vi "Pump Status.vi"(8 "error in (no error)":errorcluster, 11 "State in":T1={"State"=enum."Idle", "Start Time"=timestamp(0 s since 1904-01-01), "Configuration"={"Cycle Period"=0.0, "Ismatech"={"VISA resource name"="", "Simulated?"=FALSE, "Pump Number"=1.0, "Reverse?"=FALSE}, "Masterflex"={"VISA resource name"="", "Simulated?"=FALSE, "Pump Number"=1.0, "Reverse?"=FALSE}, "Mettler"={"VISA resource name"="", "Simulated?"=FALSE}, "Bronkhorst M13 Flow Meter"={"VISA resource name"="", "Simulated?"=FALSE, "Smoothing Steps"=1}, "PID 2 Parameters"={"Input Device"=enum."Bronkhorst M13", "Output Device"=enum."Ismatec ISM 831C", "Setpoint"=0.0, "PID gains"={"proportional gain (Kc)"=1.0, "integral time (Ti, min)"=0.01, "derivative time (Td, min)"=0.0}}, "Manual Entry"=0.0, "Auto?"=TRUE, "PID range"={"PID High"=100.0, "PID Low"=0.0, "High Warning"=100.0}, "Tacmina Settings"={"Analog DAQ Task"="", "Digital DAQ Task"=""}, "KNF SIMDOS Settings"={"VISA resource name"="", "Simulated?"=TRUE}, "ASIA Pump C"={"ASIA Pump #"=0, "channel"=0, "Simulated"=FALSE}, "VICI Settings"={"VISA resource name"="", "Pump ID"="", "Pump Head Vol"=0.0, "Reverse?"=FALSE, "Simulated?"=FALSE}, "FLOM Settings"={"VISA resource name"="", "Simulated?"=TRUE, "Pump Number"=0.0}, "SSI PR/LD Settings"={"VISA resource name"="", "Simulated?"=FALSE}, "Masterflex 75211 Settings"={"Analog DAQ Task"="", "Digital DAQ Task"=""}, "SSI P40 Settings"={"VISA resource name"="", "Simulated?"=TRUE}, "Ismatech 3 Channel Settings"={"VISA resource name"="", "Pump Number"=1, "Channel Number"=0, "Simulated?"=TRUE, "Reverse?"=FALSE}, "Bronkhorst M14 Settings"={"VISA resource name"="", "Simulated?"=FALSE, "Smoothing Steps"=1}, "Reset Totalizer"=FALSE, "Input Num Alarm Settings"=[], "Control Type"=enum."g/min", "Front End Display Options"={"Temperature"=TRUE, "Scale Grams"=FALSE, "Density"=TRUE, "Flow (g/min)"=FALSE, "Flow (ml/min)"=TRUE, "PSIG"=TRUE, "Total Grams"=TRUE, "Updated"=TRUE}}, "Current Time"=timestamp(0 s since 1904-01-01), "PID 1 Parameters"={"Setpoint"=0.0, "PID gains"={"proportional gain (Kc)"=1.0, "integral time (Ti, min)"=0.01, "derivative time (Td, min)"=0.0}}, "First Iteration"=FALSE, "Data"={"Flowmeter (g/min)"=0.0, "Flowmeter (ml/min)"=0.0, "Density"=0.0, "FL Temp"=0.0, "Scale Output (g)"=0.0, "Scale Rate of Change (g/min)"=0.0, "PID 1 Output"=0.0, "PID 2 Process Variable"=0.0, "PID 2 output"=0.0, "Pump Flow"=0.0, "Pump Pressure"=0.0, "Totalized Value"=0.0}, "Process Name"="", "Pump On?"=enum."Off", "Input Error"=FALSE, "Output Error"=FALSE, "Log Started"=FALSE, "PID Overshoot"=FALSE, "Current Setpoint"=0.0} {"PID 1 Parameters"."PID gains"."derivative time (Td, min)" format="%.3f"; "PID 1 Parameters"."PID gains"."integral time (Ti, min)" format="%.3f"; "PID 1 Parameters"."PID gains"."proportional gain (Kc)" format="%.3f"; "Configuration"."Bronkhorst M14 Settings"."Smoothing Steps" min=1 step=1; "Configuration"."Ismatech 3 Channel Settings"."Channel Number" min=0 max=3; "Configuration"."Ismatech 3 Channel Settings"."Pump Number" min=1; "Configuration"."PID range"."PID Low" min=0.0 max=100.0 format="%.2f"; "Configuration"."PID range"."PID High" format="%.2f"; "Configuration"."PID 2 Parameters"."PID gains"."derivative time (Td, min)" format="%.3f"; "Configuration"."PID 2 Parameters"."PID gains"."integral time (Ti, min)" format="%.3f"; "Configuration"."PID 2 Parameters"."PID gains"."proportional gain (Kc)" format="%.3f"; "Configuration"."Bronkhorst M13 Flow Meter"."Smoothing Steps" min=1 step=1; "Configuration"."ASIA Pump C"."channel" min=0 max=1 step=1; "Configuration"."Ismatech"."Pump Number" min=1.0 max=20.0 step=1.0; "Configuration"."Masterflex"."Pump Number" min=1.0 max=20.0 step=1.0}) -> (0 "error out":errorcluster, 3 "State out":T1={"State"=enum."Idle", "Start Time"=timestamp(0 s since 1904-01-01), "Configuration"={"Cycle Period"=0.0, "Ismatech"={"VISA resource name"="", "Simulated?"=FALSE, "Pump Number"=1.0, "Reverse?"=FALSE}, "Masterflex"={"VISA resource name"="", "Simulated?"=FALSE, "Pump Number"=1.0, "Reverse?"=FALSE}, "Mettler"={"VISA resource name"="", "Simulated?"=FALSE}, "Bronkhorst M13 Flow Meter"={"VISA resource name"="", "Simulated?"=FALSE, "Smoothing Steps"=1}, "PID 2 Parameters"={"Input Device"=enum."Bronkhorst M13", "Output Device"=enum."Ismatec ISM 831C", "Setpoint"=0.0, "PID gains"={"proportional gain (Kc)"=1.0, "integral time (Ti, min)"=0.01, "derivative time (Td, min)"=0.0}}, "Manual Entry"=0.0, "Auto?"=TRUE, "PID range"={"PID High"=100.0, "PID Low"=0.0, "High Warning"=100.0}, "Tacmina Settings"={"Analog DAQ Task"="", "Digital DAQ Task"=""}, "KNF SIMDOS Settings"={"VISA resource name"="", "Simulated?"=TRUE}, "ASIA Pump C"={"ASIA Pump #"=0, "channel"=0, "Simulated"=FALSE}, "VICI Settings"={"VISA resource name"="", "Pump ID"="", "Pump Head Vol"=0.0, "Reverse?"=FALSE, "Simulated?"=FALSE}, "FLOM Settings"={"VISA resource name"="", "Simulated?"=TRUE, "Pump Number"=0.0}, "SSI PR/LD Settings"={"VISA resource name"="", "Simulated?"=FALSE}, "Masterflex 75211 Settings"={"Analog DAQ Task"="", "Digital DAQ Task"=""}, "SSI P40 Settings"={"VISA resource name"="", "Simulated?"=TRUE}, "Ismatech 3 Channel Settings"={"VISA resource name"="", "Pump Number"=1, "Channel Number"=0, "Simulated?"=TRUE, "Reverse?"=FALSE}, "Bronkhorst M14 Settings"={"VISA resource name"="", "Simulated?"=FALSE, "Smoothing Steps"=1}, "Reset Totalizer"=FALSE, "Input Num Alarm Settings"=[], "Control Type"=enum."g/min", "Front End Display Options"={"Temperature"=TRUE, "Scale Grams"=FALSE, "Density"=TRUE, "Flow (g/min)"=FALSE, "Flow (ml/min)"=TRUE, "PSIG"=TRUE, "Total Grams"=TRUE, "Updated"=TRUE}}, "Current Time"=timestamp(0 s since 1904-01-01), "PID 1 Parameters"={"Setpoint"=0.0, "PID gains"={"proportional gain (Kc)"=1.0, "integral time (Ti, min)"=0.01, "derivative time (Td, min)"=0.0}}, "First Iteration"=FALSE, "Data"={"Flowmeter (g/min)"=0.0, "Flowmeter (ml/min)"=0.0, "Density"=0.0, "FL Temp"=0.0, "Scale Output (g)"=0.0, "Scale Rate of Change (g/min)"=0.0, "PID 1 Output"=0.0, "PID 2 Process Variable"=0.0, "PID 2 output"=0.0, "Pump Flow"=0.0, "Pump Pressure"=0.0, "Totalized Value"=0.0}, "Process Name"="", "Pump On?"=enum."Off", "Input Error"=FALSE, "Output Error"=FALSE, "Log Started"=FALSE, "PID Overshoot"=FALSE, "Current Setpoint"=0.0} {"PID 1 Parameters"."PID gains"."derivative time (Td, min)" format="%.3f"; "PID 1 Parameters"."PID gains"."integral time (Ti, min)" format="%.3f"; "PID 1 Parameters"."PID gains"."proportional gain (Kc)" format="%.3f"; "Configuration"."Bronkhorst M14 Settings"."Smoothing Steps" min=1 step=1; "Configuration"."Ismatech 3 Channel Settings"."Channel Number" min=0 max=3; "Configuration"."Ismatech 3 Channel Settings"."Pump Number" min=1; "Configuration"."PID range"."PID Low" min=0.0 max=100.0 format="%.2f"; "Configuration"."PID range"."PID High" format="%.2f"; "Configuration"."PID 2 Parameters"."PID gains"."derivative time (Td, min)" format="%.3f"; "Configuration"."PID 2 Parameters"."PID gains"."integral time (Ti, min)" format="%.3f"; "Configuration"."PID 2 Parameters"."PID gains"."proportional gain (Kc)" format="%.3f"; "Configuration"."Bronkhorst M13 Flow Meter"."Smoothing Steps" min=1 step=1; "Configuration"."ASIA Pump C"."channel" min=0 max=1 step=1; "Configuration"."Ismatech"."Pump Number" min=1.0 max=20.0 step=1.0; "Configuration"."Masterflex"."Pump Number" min=1.0 max=20.0 step=1.0})   [LabVIEW 2018]
uses:
  Measure Instrument/State Cluster.ctl
  Measure Instrument/State Enum.ctl
  Feed Module/Controls/Feed Module Settings Cluster.ctl
  Ismatec ISM 831C/Controls/Ismatech ISM831C Settings Cluster.ctl
  Masterflex 7550-30/Controls/Settings Cluster.ctl
  Mettler Toledo/Controls/Settings Cluster.ctl
  Bronkhorst M13 Flow Meter/Settings Cluster.ctl
  Measure Instrument/PID 2 Parameters Cluster.ctl
  Measure Instrument/PID Input Enum.ctl
  Measure Instrument/PID 2 Output Enum.ctl
  Tacmina QI/Tacmina QI DAQ Setting.ctl
  KNF Pump/Settings Cluster plus SIMDOS.ctl
  ASIA Pump/Pump Settings.ctl
  VICI M50 Party Mode/Settings Cluster.ctl
  FLOM Pump/Settings Cluster.ctl
  SSI PR Class/SSI PR or LD Settings Cluster.ctl
  Masterflex 75211/Masterflex 75211 DAQ Setting.ctl
  SSI PR Class/SSI P40 Settings Cluster.ctl
  Ismatec 78001/Ismatec 4083.ctl
  Bronkhorst M14 Flow Meter/Settings Cluster.ctl
  Tag VIs/Numeric Alarm Settings Cluster.ctl
  Measure Instrument/PID 1 Parameters Cluster.ctl
  Tag VIs/Tag FGV Operation Enum.ctl
  Ismatec ISM 831C/Ismatec ISM 831C.lvlib
  Masterflex 7550-30/Masterflex 7550-30.lvlib
  Measure Instrument/Feed Module Engine.lvlib
  Shared Variables/Dynamic Shared Variables.lvlib
  Tacmina QI/Tacmina QI.lvlib
  KNF Pump/KNF SIMDOS.lvlib
  ASIA Pump.lvlib
  VICI M50 Party Mode/VICI M6 M50 Party Mode.lvlib
  FLOM Pump/FLOM Pump.lvlib
  SSI PR Class/SSI PR or LD Pump.lvlib
  Ismatec 78001/Ismatec 4308.lvlib
  Mettler Toledo/Mettler Toledo.lvlib
  Bronkhorst M13 Flow Meter/Bronkhorst M13 Flow Meter.lvlib
  Feed Module/Feed Module.lvlib
  Masterflex 75211/Masterflex 75211.lvlib
  SSI PR Class/SSI P40 Pump.lvlib
  Bronkhorst M14 Flow Meter/Bronkhorst M14 Flow Meter.lvlib
panel:
  # "Output Instruments"
  # "Input Instruments"
  # "Output Instruments"
  # "Input Instruments"
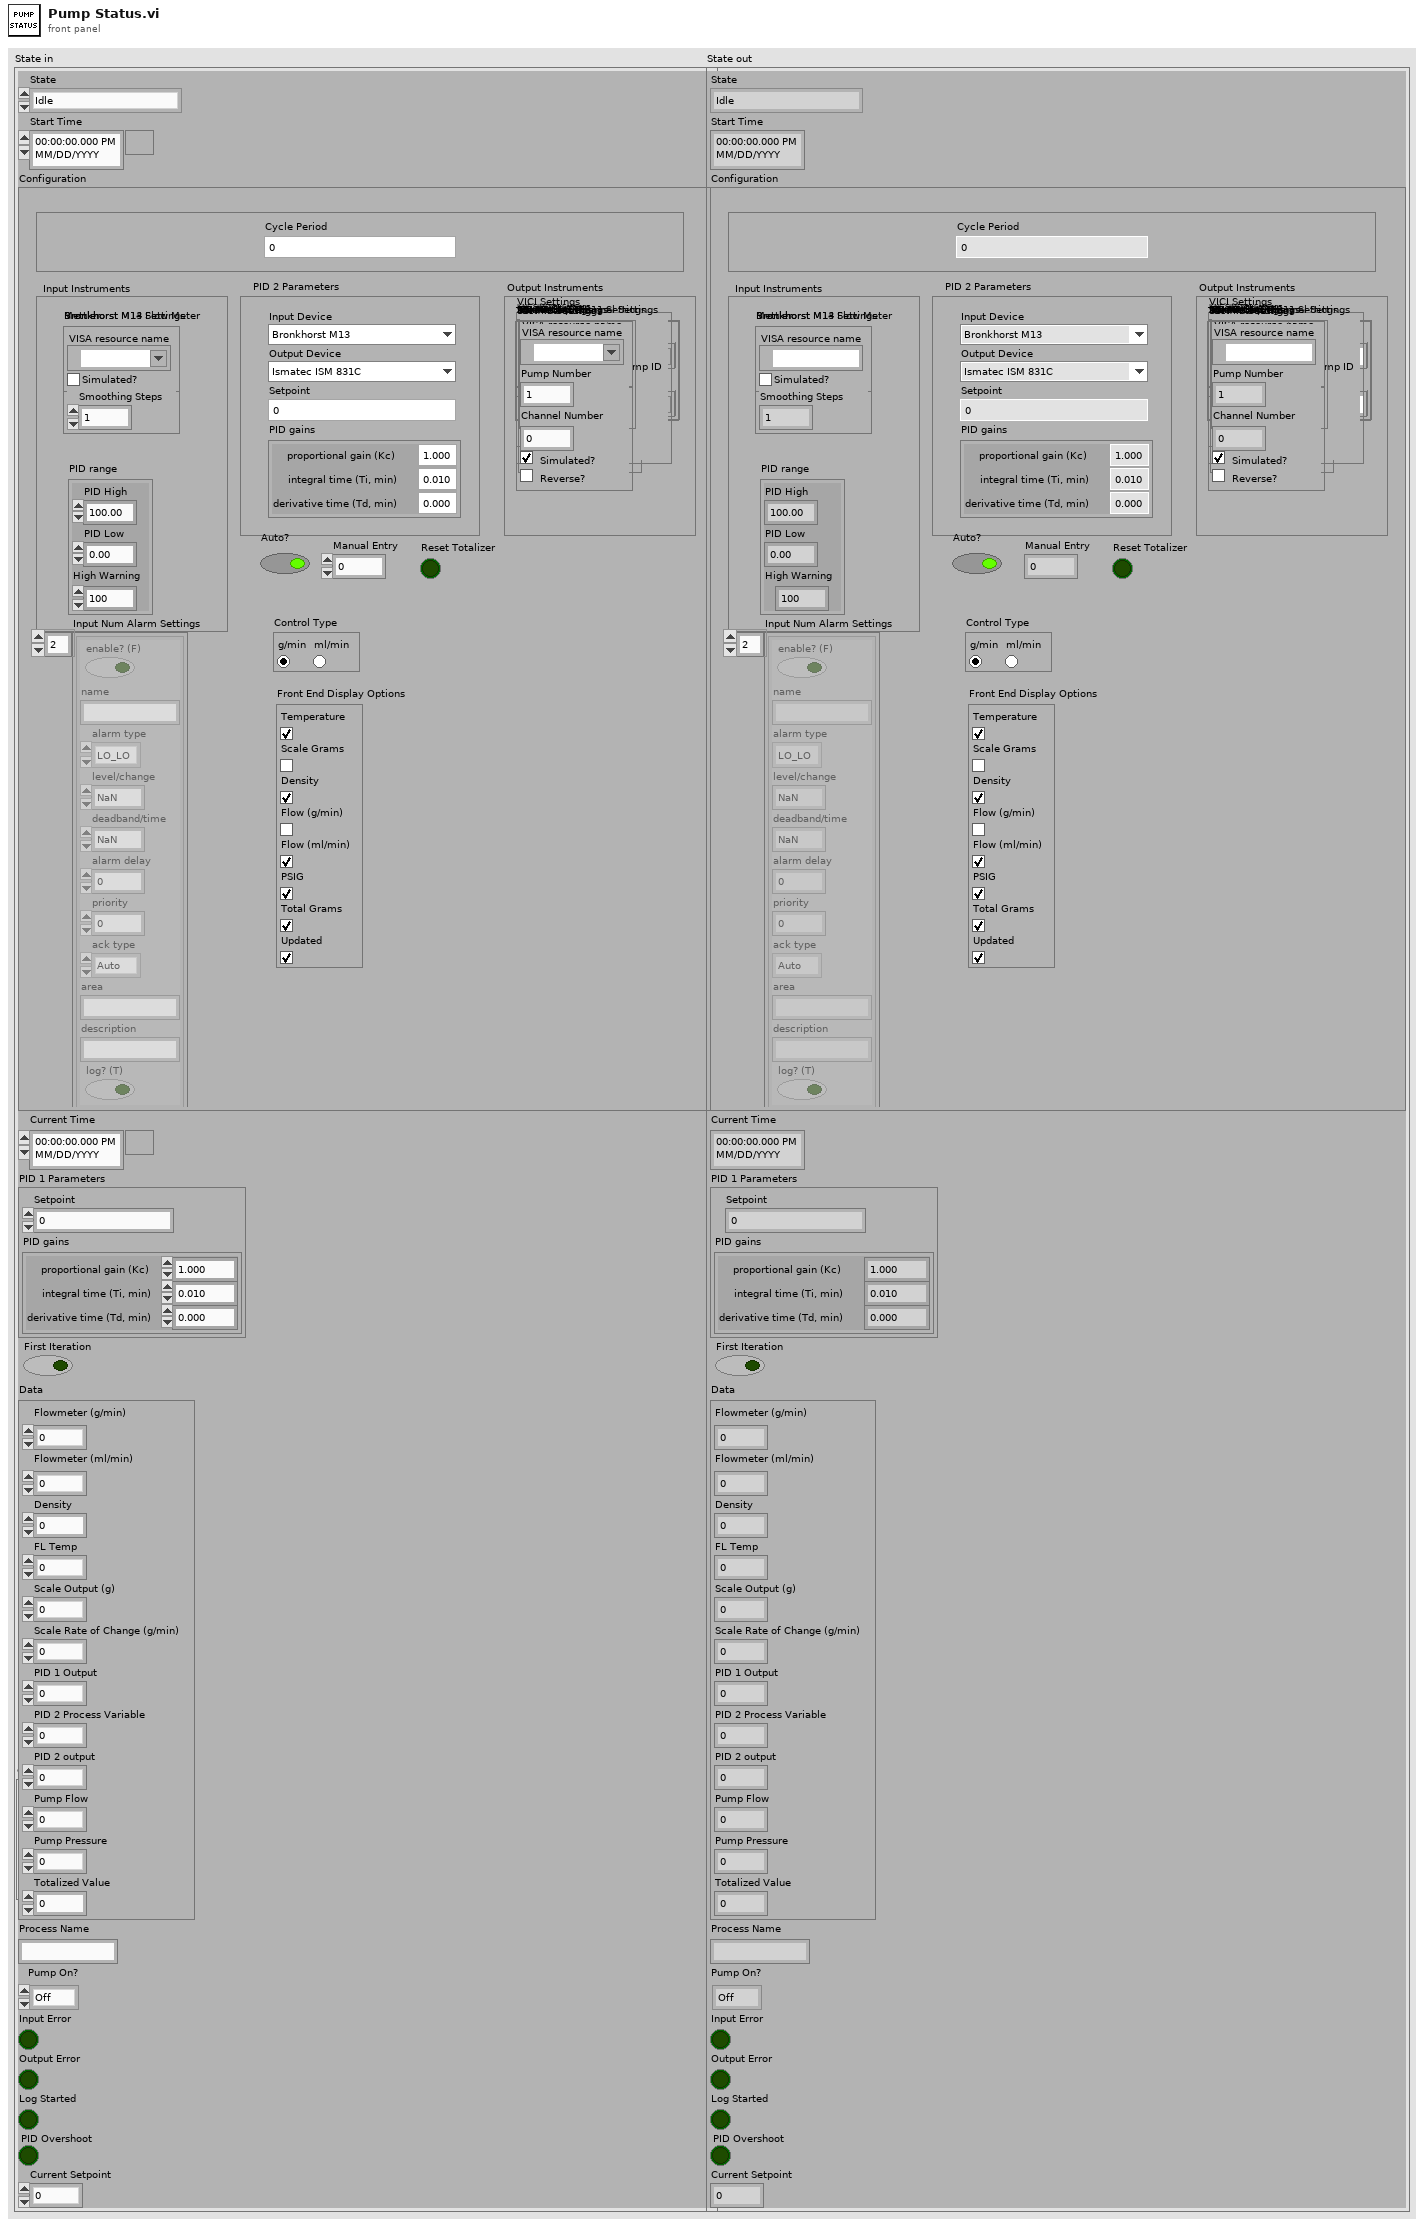
[diagram p1: front panel]
types:
  T1 = typedef "Feed Module.lvlib/Feed Module Engine.lvlib/State Cluster.ctl" = cluster{"State":T2, "Start Time":timestamp, "Configuration":T3, "Current Time":timestamp, "PID 1 Parameters":T22, "First Iteration":bool, "Data":cluster{"Flowmeter (g/min)":dbl, "Flowmeter (ml/min)":dbl, "Density":dbl, "FL Temp":dbl, "Scale Output (g)":dbl, "Scale Rate of Change (g/min)":dbl, "PID 1 Output":dbl, "PID 2 Process Variable":dbl, "PID 2 output":dbl, "Pump Flow":dbl, "Pump Pressure":dbl, "Totalized Value":dbl}, "Process Name":string, "Pump On?":enum16{"Off", "On", "Not Initialized"}, "Input Error":bool, "Output Error":bool, "Log Started":bool, "PID Overshoot":bool, "Current Setpoint":dbl}
  T2 = typedef "Feed Module.lvlib/Feed Module Engine.lvlib/State Enum.ctl" = enum16{"Measuring", "Idle", "Paused"}
  T3 = typedef "Feed Module.lvlib/Feed Module Settings Cluster.ctl" = cluster{"Cycle Period":dbl, "Ismatech":T4, "Masterflex":T5, "Mettler":T6, "Bronkhorst M13 Flow Meter":T7, "PID 2 Parameters":T8, "Manual Entry":dbl, "Auto?":bool, "PID range":cluster{"PID High":dbl, "PID Low":dbl, "High Warning":dbl}, "Tacmina Settings":T11, "KNF SIMDOS Settings":T12, "ASIA Pump C":T13, "VICI Settings":T14, "FLOM Settings":T15, "SSI PR/LD Settings":T16, "Masterflex 75211 Settings":T17, "SSI P40 Settings":T18, "Ismatech 3 Channel Settings":T19, "Bronkhorst M14 Settings":T20, "Reset Totalizer":bool, "Input Num Alarm Settings":T21[], "Control Type":enum32{"g/min", "ml/min"}, "Front End Display Options":cluster{"Temperature":bool, "Scale Grams":bool, "Density":bool, "Flow (g/min)":bool, "Flow (ml/min)":bool, "PSIG":bool, "Total Grams":bool, "Updated":bool}}
  T4 = typedef "Ismatec ISM 831C.lvlib/Ismatech ISM831C Settings Cluster.ctl" = cluster{"VISA resource name":refnum<visa-resource-name>, "Simulated?":bool, "Pump Number":dbl, "Reverse?":bool}
  T5 = typedef "Masterflex 7550-30.lvlib/Settings Cluster.ctl" = cluster{"VISA resource name":refnum<visa-resource-name>, "Simulated?":bool, "Pump Number":dbl, "Reverse?":bool}
  T6 = typedef "Mettler Toledo.lvlib/Settings Cluster.ctl" = cluster{"VISA resource name":refnum<visa-resource-name>, "Simulated?":bool}
  T7 = typedef "Bronkhorst M13 Flow Meter.lvlib/Settings Cluster.ctl" = cluster{"VISA resource name":refnum<visa-resource-name>, "Simulated?":bool, "Smoothing Steps":i32}
  T8 = typedef "PID 2 Parameters Cluster.ctl" = cluster{"Input Device":T9, "Output Device":T10, "Setpoint":dbl, "PID gains":cluster{"proportional gain (Kc)":dbl, "integral time (Ti, min)":dbl, "derivative time (Td, min)":dbl}}
  T9 = typedef "PID Input Enum.ctl" = enum16{"Default", "Bronkhorst M13", "Bronkhorst M14", "Scale Rate of Change"}
  T10 = typedef "PID 2 Output Enum.ctl" = enum16{"Default", "Ismatec ISM 4308", "Ismatec ISM 831C", "Masterflex 7550-30", "VICI M6", "VICI M50", "Tacmina QI", "KNF SIMDOS", "ASIA Type C", "FLOM UI-22-11", "SSI PR/LD", "SSI P40", "Masterflex 75211-70"}
  T11 = typedef "Tacmina QI.lvlib/Tacmina QI DAQ Setting.ctl" = cluster{"Analog DAQ Task":refnum<k21>, "Digital DAQ Task":refnum<k21>}
  T12 = typedef "KNF SIMDOS.lvlib/Settings Cluster plus SIMDOS.ctl" = cluster{"VISA resource name":refnum<visa-resource-name>, "Simulated?":bool}
  T13 = typedef "ASIA Pump.lvlib/Pump Settings.ctl" = cluster{"ASIA Pump #":i32, "channel":i32, "Simulated":bool}
  T14 = typedef "VICI M6 M50 Party Mode.lvlib/Settings Cluster.ctl" = cluster{"VISA resource name":refnum<visa-resource-name>, "Pump ID":string, "Pump Head Vol":dbl, "Reverse?":bool, "Simulated?":bool}
  T15 = typedef "FLOM Pump.lvlib/Settings Cluster.ctl" = cluster{"VISA resource name":refnum<visa-resource-name>, "Simulated?":bool, "Pump Number":dbl}
  T16 = typedef "SSI PR or LD Pump.lvlib/SSI PR or LD Settings Cluster.ctl" = cluster{"VISA resource name":refnum<visa-resource-name>, "Simulated?":bool}
  T17 = typedef "Masterflex 75211.lvlib/Masterflex 75211 DAQ Setting.ctl" = cluster{"Analog DAQ Task":refnum<k21>, "Digital DAQ Task":refnum<k21>}
  T18 = typedef "SSI P40 Pump.lvlib/SSI P40 Settings Cluster.ctl" = cluster{"VISA resource name":refnum<visa-resource-name>, "Simulated?":bool}
  T19 = typedef "Ismatec 4308.lvlib/Ismatec 4083.ctl" = cluster{"VISA resource name":refnum<visa-resource-name>, "Pump Number":i16, "Channel Number":i16, "Simulated?":bool, "Reverse?":bool}
  T20 = typedef "Bronkhorst M14 Flow Meter.lvlib/Settings Cluster.ctl" = cluster{"VISA resource name":refnum<visa-resource-name>, "Simulated?":bool, "Smoothing Steps":i32}
  T21 = typedef "Numeric Alarm Settings Cluster.ctl" = cluster{"enable? (F)":bool, "name":string, "alarm type":enum16{"HI_HI", "HI", "LO", "LO_LO"}, "level/change":dbl, "deadband/time":dbl, "alarm delay":dbl, "priority":u32, "ack type":enum16{"Auto", "User", "None", "Each Occurrence"}, "area":string, "description":string, "log? (T)":bool}
  T22 = typedef "PID 1 Parameters Cluster.ctl" = cluster{"Setpoint":dbl, "PID gains":cluster{"proportional gain (Kc)":dbl, "integral time (Ti, min)":dbl, "derivative time (Td, min)":dbl}}
  T23 = typedef "Tag FGV Operation Enum.ctl" = enum16{"Init", "Set Notification Queue", "Create Tag", "Commit", "Write Tag (Numeric)", "Write Tag (Boolean)", "Read All Tags", "Read One Tag", "Delete Tag Category", "Set Alarm Parameters (Numeric)", "Set Alarm Parameters (Boolean)", "Enable All Alarms", "Disable All Alarms", "Delete All Tags", "Read Alarms", "Ack Alarm", "Read Alarm Parameters (Numeric)", "Read Alarm Parameters (Boolean)"}
  T24 = typedef "Feed Module.lvlib/Feed Module Tag Names Cluster.ctl" = cluster{"Pump Flow g Tag":string, "PID 2 Out Tag":string, "Totalized Tag":string, "Pump Flow ml Tag":string, "Identifier Tag":string, "Scale Tag":string, "Density Tag":string, "FL Temp":string, "Input Device Tag":string, "Output Device Tag":string, "Pump's Flow":string, "Pump's Pressure":string, "Overpressure Tag":string}
  T25 = cluster{"alarm URL":string, "set time":timestamp, "set user":string, "ack time":timestamp, "ack user":string, "clear time":timestamp, "clear user":string, "setpoint":dbl, "value":dbl, "priority":u32, "alarm area":string, "alarm description":string, "ack comment":string, "event?":bool, "Refnum":u64}[]
  T26 = typedef "Dynamic Shared Variables.lvlib/Alarm Cluster (UI).ctl" = cluster{"Color Box":u32, "Name":string, "Ack":bool}
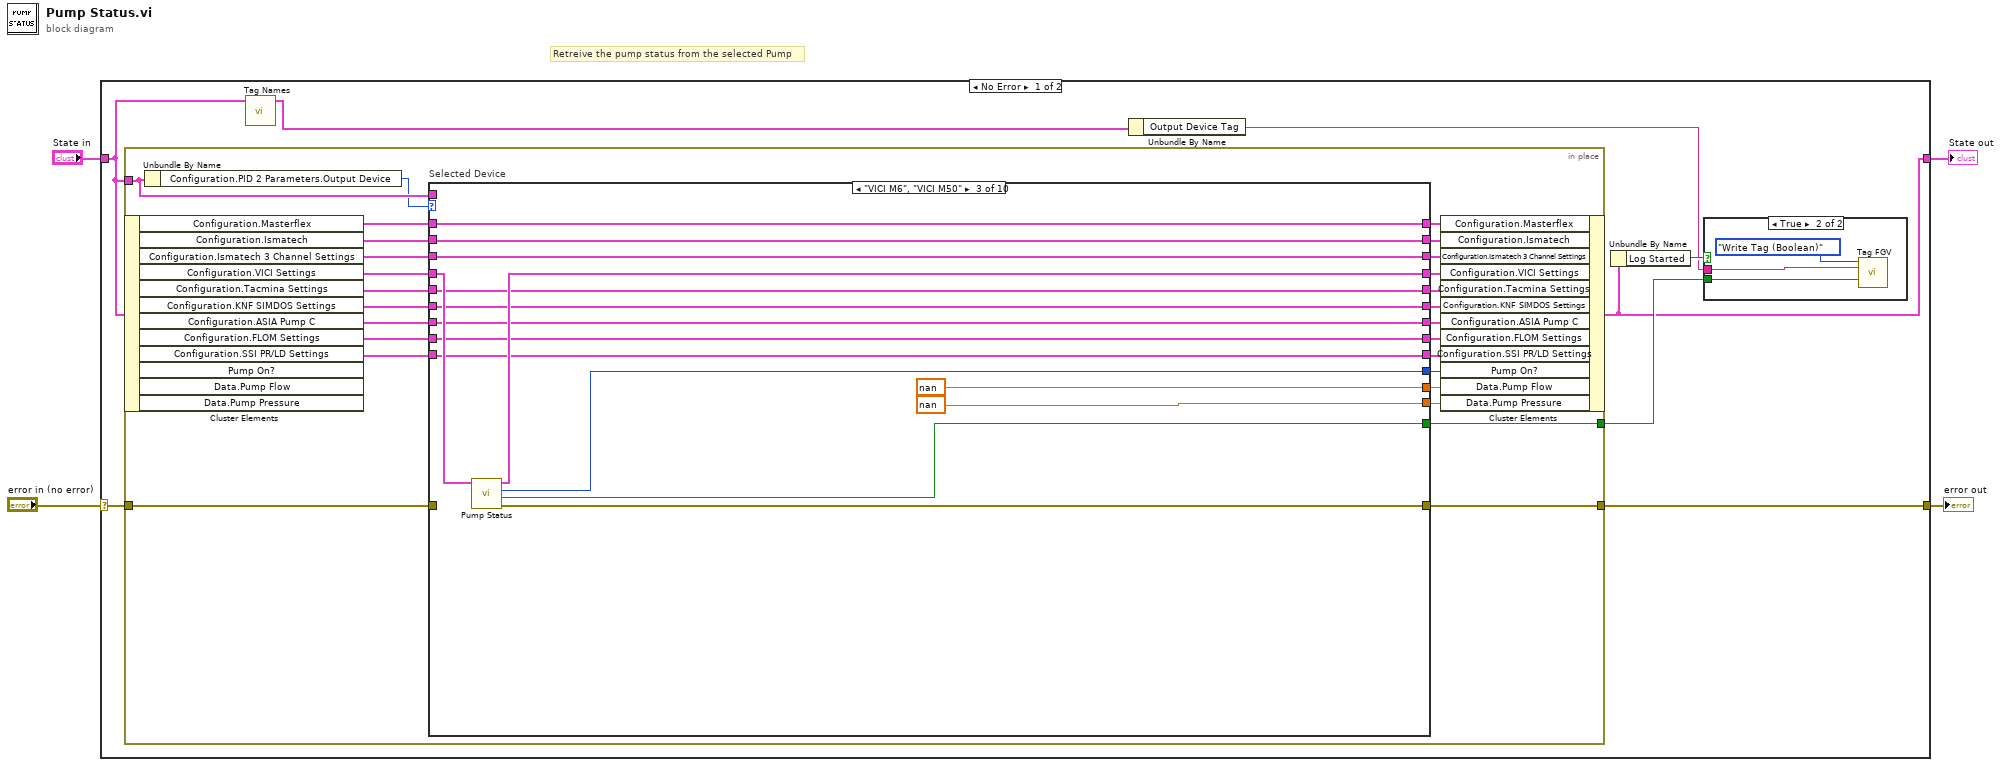
[diagram p0: block diagram]
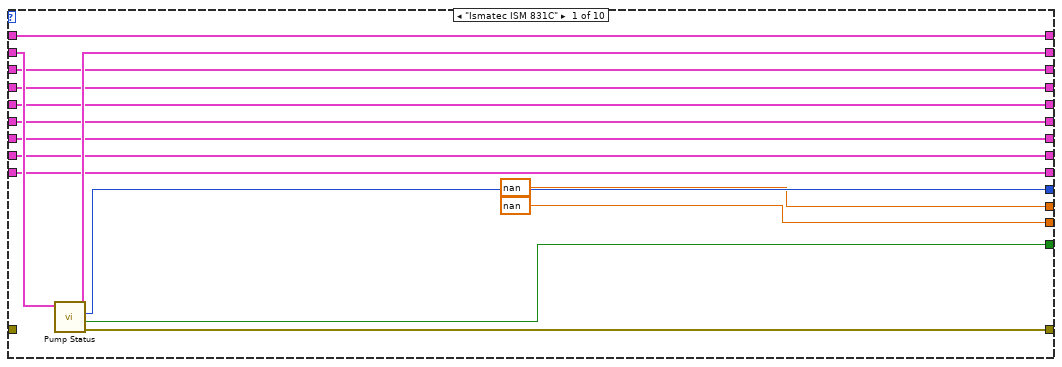
[diagram p2: hidden frame]
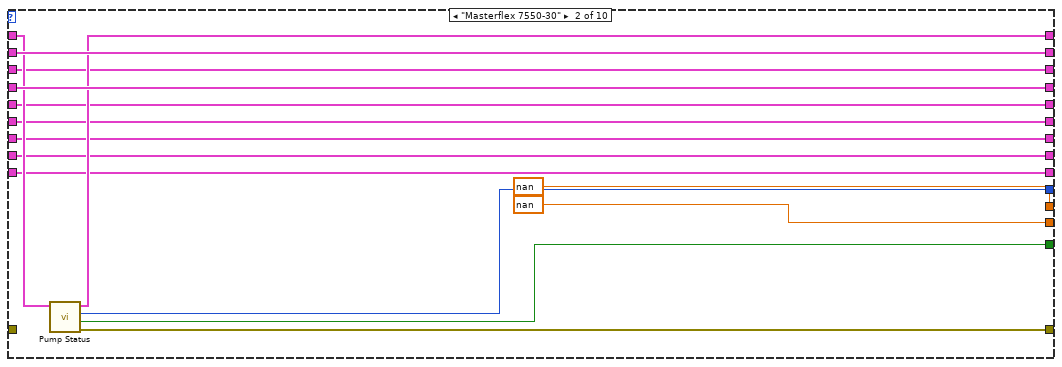
[diagram p3: hidden frame]
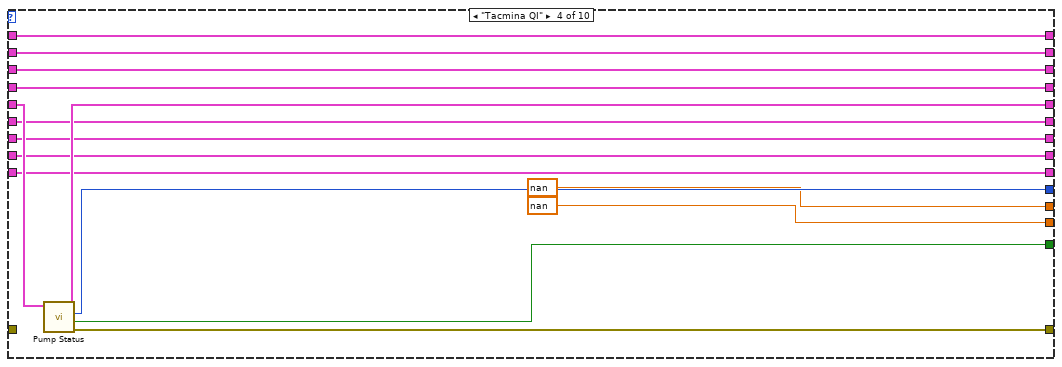
[diagram p4: hidden frame]
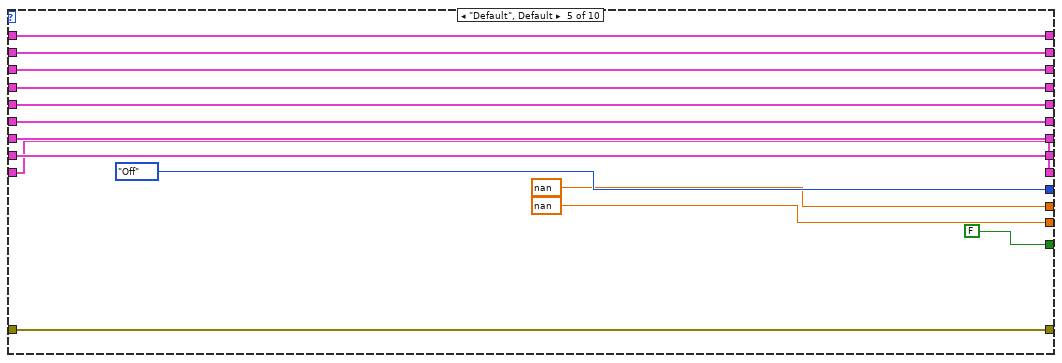
[diagram p5: hidden frame]
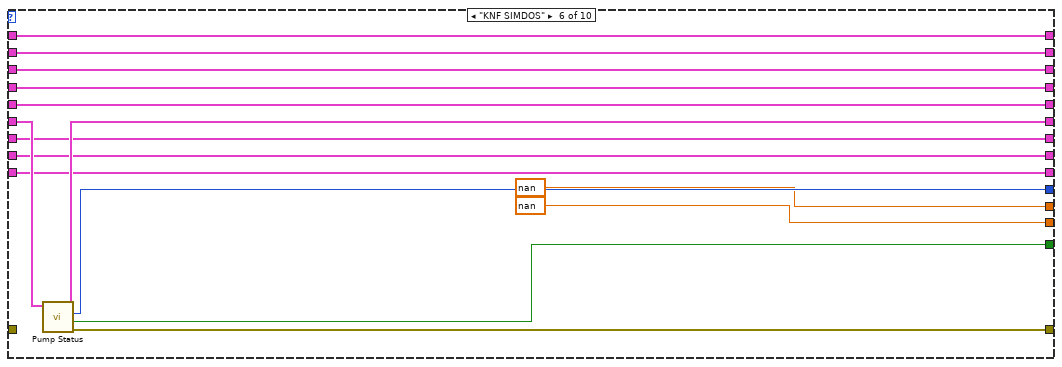
[diagram p6: hidden frame]
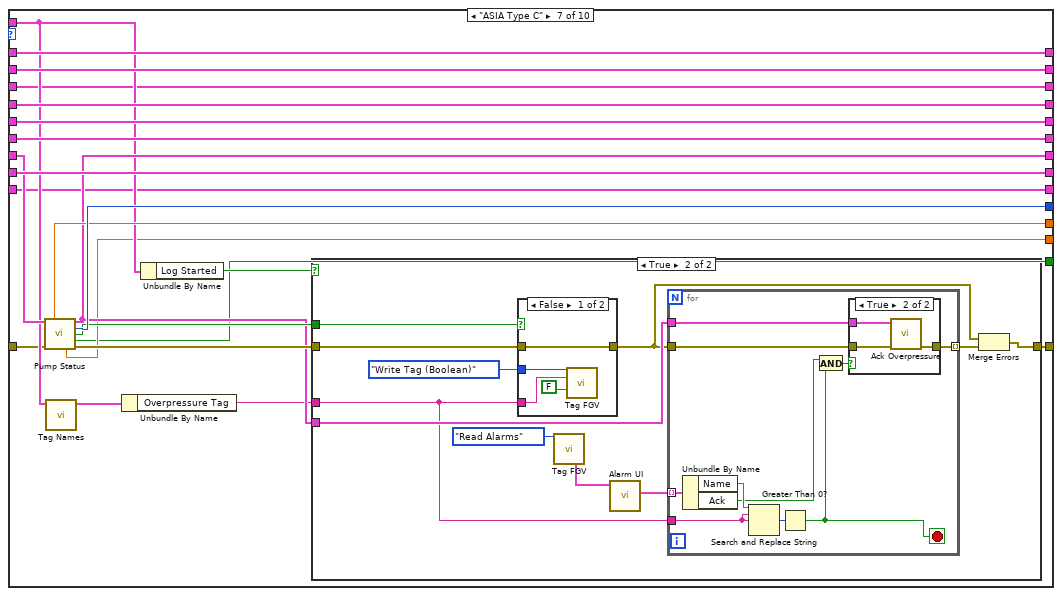
[diagram p7: hidden frame]
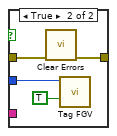
[diagram p10: hidden frame]
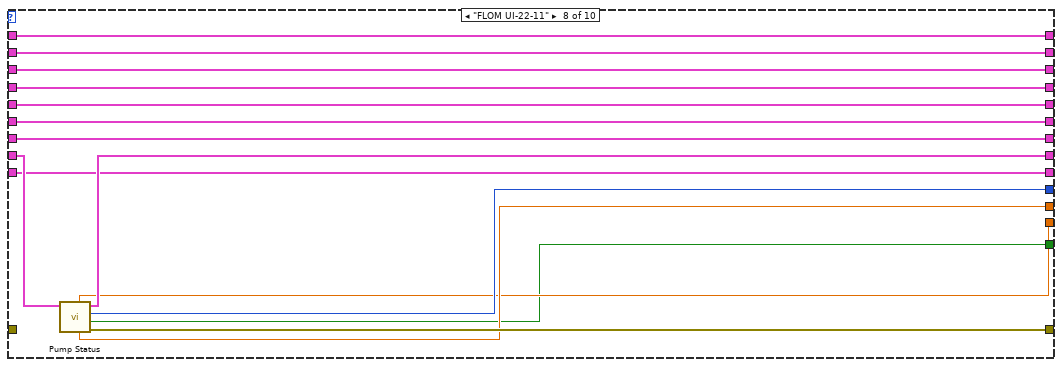
[diagram p11: hidden frame]
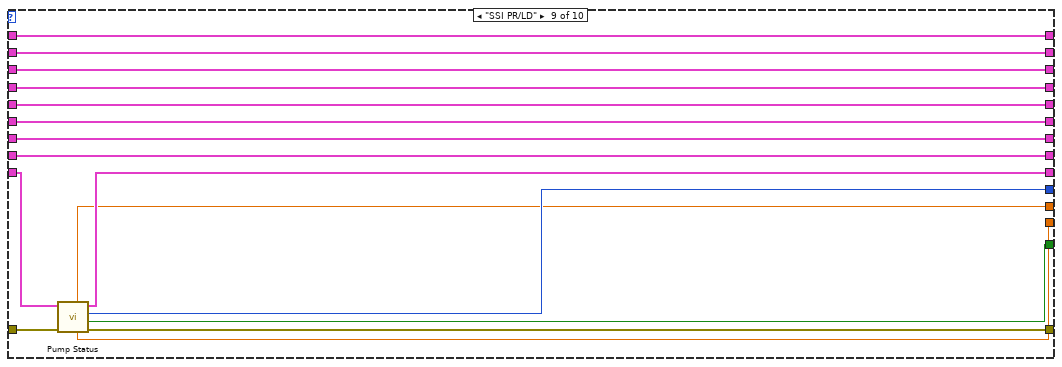
[diagram p12: hidden frame]
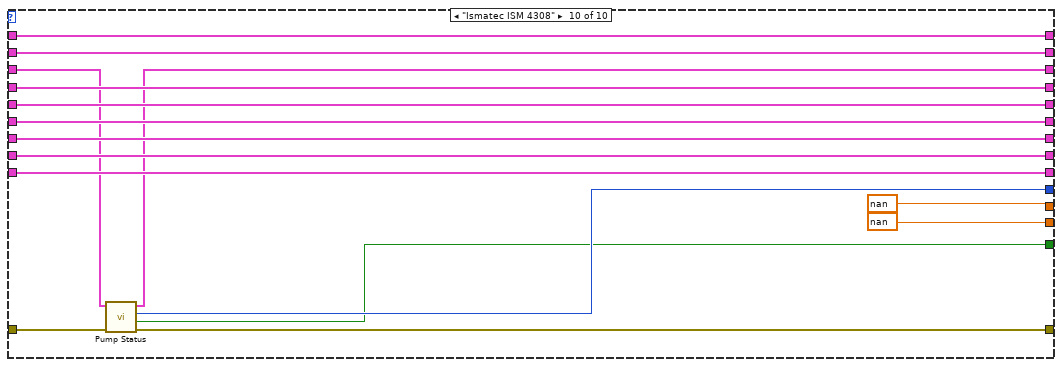
[diagram p13: hidden frame]
diagram:
  # "Retreive the pump status from the selected Pump"
  n1 = case shown="No Error" "error in (no error)" {
    selector: "error in (no error)" -> [w10 w235]
    tunnel: [w11 w235] -> w3
    tunnel: "State in" -> [w6 w234]
    tunnel: [w5 w234] -> w1
    frame No Error {
      n2 = in-place {
        in-place-border: w6 -> [w38]
        in-place-border: [w37] -> w11
        in-place-border: w10 -> [w36]
        in-place-border: [w35] -> w9
        n3 = in-place-cluster #1(w6) -> ("Configuration.Masterflex"=w33:T5, "Configuration.Ismatech"=w32:T4, "Configuration.Ismatech 3 Channel Settings"=w13:T19, "Configuration.VICI Settings"=w31:T14, "Configuration.Tacmina Settings"=w30:T11, "Configuration.KNF SIMDOS Settings"=w29:T12, "Configuration.ASIA Pump C"=w28:T13, "Configuration.FLOM Settings"=w27:T15, "Configuration.SSI PR/LD Settings"=w26:T16)  [unwired: 3 out]
        n4 = Unbundle By Name(w38) -> ("Configuration.PID 2 Parameters.Output Device"=w34:T10)
        n5 = case "Selected Device" shown="\"VICI M6\", \"VICI M50\"" w34 {
          tunnel: w33 -> [w53 w64 w82 w98 w112 w127 w149 w198 w204 w220]
          tunnel: [w53 w65 w82 w98 w112 w127 w149 w198 w204 w220] -> w25
          tunnel: w32 -> [w51 w68 w83 w97 w111 w126 w148 w197 w214 w230]
          tunnel: [w52 w66 w79 w94 w102 w123 w137 w192 w206 w217] -> w37
          tunnel: w36 -> [_ _ _ _ w102 _ w134 _ w207 w223]
          tunnel: [w50 w68 w83 w97 w111 w126 w148 w197 w214 w230] -> w24
          tunnel: w31 -> [w48 w67 w80 w96 w110 w125 w147 w196 w213 w229]
          tunnel: [w48 w67 w81 w96 w110 w125 w147 w196 w213 w229] -> w23
          tunnel: w30 -> [w49 w63 w78 w95 w109 w124 w146 w195 w212 w228]
          tunnel: [w49 w63 w78 w93 w109 w124 w146 w195 w212 w228] -> w22
          tunnel: [w47 w62 w77 w92 w108 w122 w145 w194 w211 w227] -> w21
          tunnel: w29 -> [w47 w62 w77 w92 w108 w121 w145 w194 w211 w227]
          tunnel: [w46 w60 w76 w91 enum16{"Off", "On", "Not Initialized"}."Off" ("Pump On?") w120 w142 w189 w203 w219] -> w17
          tunnel: [w45 w61 w75 w90 w106 w119 w136 w193 w210 w226] -> w20
          tunnel: w28 -> [w45 w61 w75 w90 w106 w119 w143 w193 w210 w226]
          tunnel: [w44 w59 w74 w89 w105 w118 w144 w191 w209 w225] -> w19
          tunnel: w27 -> [w44 w59 w74 w89 w105 w118 w144 w190 w209 w225]
          tunnel: [nan ("Pressure") nan ("Pressure") nan ("Pressure") nan ("Pressure") nan ("Pressure") nan ("Pressure") w140 w188 w202 nan ("Pressure")] -> w16
          tunnel: w38 -> [_ _ _ _ _ _ w135 _ _ _]
          tunnel: [nan ("Flow Rate") nan ("Flow Rate") nan ("Flow Rate") nan ("Flow Rate") nan ("Flow Rate") nan ("Flow Rate") w133 w187 w201 nan ("Flow Rate")] -> w15
          tunnel: [w41 w56 w71 w86 FALSE ("Connection Error") w115 w132 w186 w200 w218] -> w35
          tunnel: w26 -> [w40 w55 w70 w85 w100 w114 w129 w185 w208 w224]
          tunnel: [w40 w55 w70 w85 w100 w114 w129 w185 w205 w224] -> w18
          tunnel: [w39 w54 w69 w84 w99 w113 w128 w184 w199 w221] -> w14
          tunnel: w13 -> [w39 w54 w69 w84 w99 w113 w128 w184 w199 w222]
          frame "Ismatec ISM 831C" {
            n6 = call "Pump Status.vi"("Ismatech Settings In"=w51) -> ("error out"=w52:errorcluster, "Connection Error"=w41:bool, "Pump On?"=w46:enum16{"Off", "On", "Not Initialized"}, "Ismatech Settings Out"=w50:T4)  [unwired: 7 in]
          }
          frame "Masterflex 7550-30" {
            n7 = call "Pump Status.vi"("Masterflex Settings in"=w64) -> ("error out"=w66:errorcluster, "Connection Error"=w56:bool, "Pump On?"=w60:enum16{"Off", "On", "Not Initialized"}, "Masterflex Settings out"=w65:T5)  [unwired: 7 in]
          }
          frame "VICI M6", "VICI M50" {
            n8 = call "Pump Status.vi"("VICI Settings In"=w80) -> ("error out"=w79:errorcluster, "Connection Error"=w71:bool, "Pump On?"=w76:enum16{"Off", "On", "Not Initialized"}, "VICI Settings Out"=w81:T14)  [unwired: 7 in]
          }
          frame "Tacmina QI" {
            n9 = call "Pump Status.vi"("Tacmina Settings in"=w95) -> ("error out"=w94:errorcluster, "Connection Error"=w86:bool, "Pump On?"=w91:enum16{"Off", "On", "Not Initialized"}, "Tacmina Settings out"=w93:T11)  [unwired: 7 in]
          }
          frame "Default", Default {
          }
          frame "KNF SIMDOS" {
            n10 = call "Pump Status.vi"("KNF Settings In"=w121) -> ("error out"=w123:errorcluster, "Connection Error"=w115:bool, "Pump On?"=w120:enum16{"Off", "On", "Not Initialized"}, "KNF Settings Out"=w122:T12)  [unwired: 7 in]
          }
          frame "ASIA Type C" {
            n11 = call "Pump Status.vi"("ASIA Pump C Settings in"=w143, "error in (no error)"=w134) -> ("pressure"=w140:dbl, "ASIA Pump C Settings out"=w136:T13, "Pump On?"=w142:enum16{"Off", "On", "Not Initialized"}, "Overpressure"=w139:bool, "Connection Error"=w132:bool, "pumpRate"=w133:dbl, "error out"=w141:errorcluster)  [unwired: 5 in, 2 out]
            n12 = call "Tag Names.vi"("State in"=w135) -> ("Feed Module Tag Names"=w131:T24)  [unwired: 6 in, 4 out]
            n13 = Unbundle By Name(w131) -> ("Overpressure Tag"=w130:string)
            n14 = Unbundle By Name(w135) -> ("Log Started"=w138:bool)
            n15 = case shown="True" w138 {
              tunnel: w141 -> [w150 w161]
              tunnel: w139 -> [_ w160]
              tunnel: [w150 w152] -> w137
              tunnel: w136 -> [_ w157]
              tunnel: w130 -> [_ w156]
              frame False {
              }
              frame True {
                n16 = case shown="False" w160 {
                  tunnel: Tag_FGV_Operation_Enum."Write Tag (Boolean)" ("Operation") -> [w177 w180]
                  tunnel: [w179 w182] -> w151
                  tunnel: w161 -> [w179 w183]
                  tunnel: w156 -> [w178 _]
                  frame False {
                    n17 = call "Tag FGV.vi"("Operation"=w177, "Tag Name"=w178, "Data"=FALSE) -> ()  [unwired: 5 in, 8 out]
                  }
                  frame True {
                    n18 = call <vilib>:"Clear Errors.vi"("error in (no error)"=w183) -> ("error out"=w182:errorcluster)  [unwired: 5 in, 1 out]
                    n19 = call "Tag FGV.vi"("Operation"=w180, "Data"=TRUE) -> ()  [unwired: 6 in, 8 out]
                  }
                }
                n20 = call "Tag FGV.vi"("Operation"=Tag_FGV_Operation_Enum."Read Alarms") -> ("alarms"=w155:T25)  [unwired: 7 in, 7 out]
                n21 = call "Alarm UI.vi"("alarms"=w155) -> ("UI Alarms"=w158:T26[])  [unwired: 9 in, 1 out]
                n22 = for {
                  tunnel: w158 -> [w171] mode=indexing
                  tunnel: w157 -> [w168]
                  tunnel: [w167] -> w153 mode=indexing
                  tunnel: w151 -> [w166]
                  tunnel: w156 -> [w162]
                  stop <- w164 stop-if-true
                  n23 = Unbundle By Name(w171) -> ("Name"=w170:string, "Ack"=w163:bool)
                  n24 = Search and Replace String(input string=w170, search string=w162, replace string=w162) -> (number of replacements=w169:i32)  [unwired: 5 in, 3 out]
                  n25 = Greater Than 0?(x=w169) -> (x > 0?=w164:bool)
                  n26 = And(x=w163, y=w164) -> (x .and. y?=w165:bool)
                  n27 = case shown="True" w165 {
                    tunnel: w168 -> [_ w175]
                    tunnel: [w172 w174] -> w167
                    tunnel: w166 -> [w172 w173]
                    frame False {
                    }
                    frame True {
                      n28 = call "Ack Overpressure.vi"("error in (no error)"=w173, "ASIA Pump C Settings in"=w175) -> ("error out"=w174:errorcluster)  [unwired: 9 in]
                    }
                  }
                }
                n29 = Merge Errors(w151, w153) -> (w152:errorcluster)
              }
            }
          }
          frame "FLOM UI-22-11" {
            n30 = call "Pump Status.vi"("FLOM Settings In"=w190) -> ("error out"=w192:errorcluster, "Connection Error"=w186:bool, "Pump On?"=w189:enum16{"Off", "On", "Not Initialized"}, "FLOM Settings Out"=w191:T15, "Pressure"=w188:dbl, "Flow Rate"=w187:dbl)  [unwired: 5 in]
          }
          frame "SSI PR/LD" {
            n31 = call "Pump Status.vi"("error in (no error)"=w207, "SSI PR Settings"=w208) -> ("error out"=w206:errorcluster, "Connection Error"=w200:bool, "Pump On?"=w203:enum16{"Off", "On", "Not Initialized"}, "SSI PR Settings"=w205:T16, "Pressure"=w201:dbl, "Flow"=w202:dbl)  [unwired: 4 in]
          }
          frame "Ismatec ISM 4308" {
            n32 = call "Pump Status.vi"("error in (no error)"=w223, "Ismatech 3 Channel Settings In"=w222) -> ("error out"=w217:errorcluster, "Connection Error"=w218:bool, "Pump On?"=w219:enum16{"Off", "On", "Not Initialized"}, "Ismatech 3 Channel Settings Out"=w221:T19)  [unwired: 5 in, 1 out]
          }
        }
        n33 = in-place-cluster #1("Configuration.Masterflex"=w25, "Configuration.Ismatech"=w24, "Configuration.Ismatech 3 Channel Settings"=w14, "Configuration.VICI Settings"=w23, "Configuration.Tacmina Settings"=w22, "Configuration.KNF SIMDOS Settings"=w21, "Configuration.ASIA Pump C"=w20, "Configuration.FLOM Settings"=w19, "Configuration.SSI PR/LD Settings"=w18, "Pump On?"=w17, "Data.Pump Flow"=w16, "Data.Pump Pressure"=w15) -> (w5:T1)
      }
      n34 = call "Tag Names.vi"("State in"=w6) -> ("Feed Module Tag Names"=w8:T24)  [unwired: 6 in, 4 out]
      n35 = Unbundle By Name(w8) -> ("Output Device Tag"=w7:string)
      n36 = Unbundle By Name(w5) -> ("Log Started"=w12:bool)
      n37 = case shown="True" w12 {
        tunnel: w7 -> [_ w232]
        tunnel: w9 -> [_ w231]
        frame False {
        }
        frame True {
          n38 = call "Tag FGV.vi"("Operation"=Tag_FGV_Operation_Enum."Write Tag (Boolean)", "Tag Name"=w232, "Data"=w231) -> ()  [unwired: 5 in, 8 out]
        }
      }
    }
    frame Error {
    }
  }
  "error out" <- w3
  "State out" <- w1
